vi "SENS_OFFS_OFFS.vi"(0 "VISA IN":refnum<visa-resource-name>, 1 "Offset Frq.":i32, 5 "error in":errorcluster, 7 "Channel":i32) -> (14 "VISA Out":refnum<visa-resource-name>, 19 "error out":errorcluster)   [LabVIEW 2018, in "PNA-X.lvlib"]
doc: "SENSe<cnum>:OFFSet:OFFSet <num> \n1791\n\n(Read-Write) Specifies an absolute offset frequency in Hz. For mixer measurements, this would be \nthe LO frequency. \nParameters \n<cnum> Any existing channel number. If unspecified, value is set to 1 \n<num> Offset frequency. Range is +/- 1000 GHz. Offsets can be positive or negative \nExamples SENS:OFFS:OFFS 1GHz \nsense2:offset:offset 1e9 \nQuery Syntax SENSe<cnum>:OFFSet:OFFSet? \nReturn Type Numeric \nDefault 0 Hz"
uses:
  PNA-X.lvlib
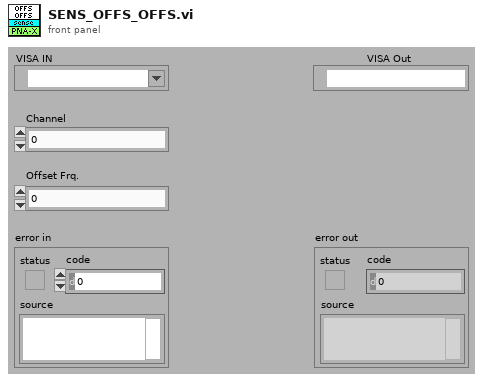
[diagram p1: front panel]
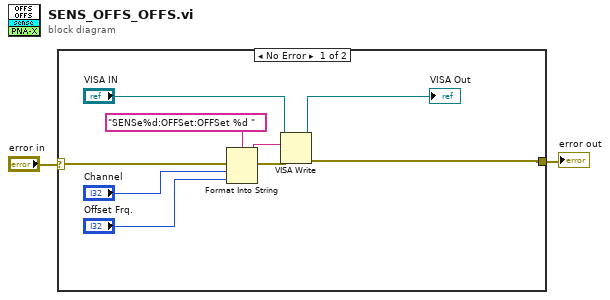
[diagram p0: block diagram]
diagram:
  n1 = case shown="No Error" "error in" {
    selector: "error in" -> [w11 w12]
    tunnel: [w6 w12] -> w1
    frame No Error {
      n2 = Format Into String(format string="SENSe%d:OFFSet:OFFSet %d " ("Cmdline"), error in=w11, "Channel", "Offset Frq.") -> (resulting string=w9:string, error out=w10:errorcluster)  [unwired: 1 in]
      n3 = VISA Write(VISA resource name="VISA IN", write buffer=w9, error in (no error)=w10) -> (VISA resource name out=→"VISA Out":refnum<visa-resource-name>, error out=w6:errorcluster)  [unwired: 1 out]
    }
    frame Error {
    }
  }
  "error out" <- w1
